vi "daqio_Write_Single.vi"(7 "daq.io Device Channel Key":string, 8 "error in (no error)":errorcluster, 9 "timestamp":timestamp, 10 "value":dbl, 11 "daq.io type in":T1={"daq.io ref"=refnum, "daq.io API Base"="http://dashboard.daq.io/api/v1", "Device Type Key"="", "Device Key"="", "Account ID"="", "online"=FALSE, "SSL"=TRUE}) -> (0 "error out":errorcluster, 3 "daq.io type out":T1={"daq.io ref"=refnum, "daq.io API Base"="http://dashboard.daq.io/api/v1", "Device Type Key"="", "Device Key"="", "Account ID"="", "online"=FALSE, "SSL"=TRUE})   [LabVIEW 2013, in "daqio minimal.lvlib"]
doc: "This VI writes a data point to a channel of a daq.io device. \n\nIf the daq.io Device Channel does not exist online, a new channel will be auto-created and data will be stored there. You have to provide a Channel Key where the value will be written to."
uses:
  daqio minimal.lvlib
  _typedefs/daqio-Type.ctl
  <vilib>/httpClient/ClientHandle.ctl
  _typedefs/daqio-TimeSeriesEntry.ctl
  _typedefs/FGV_commands.ctl
  _typedefs/daqio-Buffer-Commands.ctl
  _typedefs/connection_FGV_commands.ctl
  <vilib>/Easy HTTP Client/Easy HTTP.lvlib
  <vilib>/httpClient/LabVIEWHTTPClient.lvlib
panel:
  out "JSON string":string
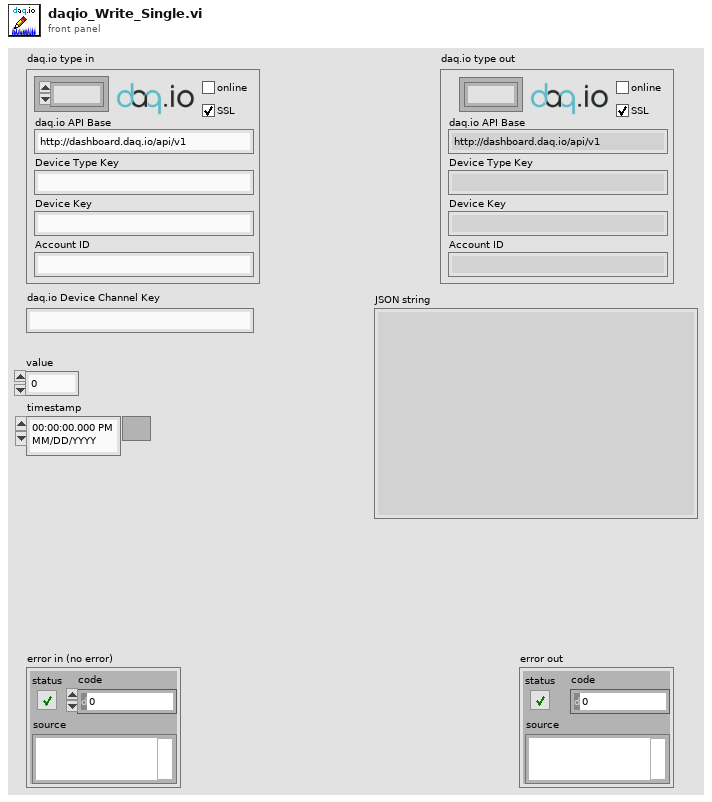
[diagram p1: front panel]
types:
  T1 = typedef "daqio minimal.lvlib/daqio-Type.ctl" = cluster{"daq.io ref":T2, "daq.io API Base":string, "Device Type Key":string, "Device Key":string, "Account ID":string, "online":bool, "SSL":bool}
  T2 = typedef "LabVIEWHTTPClient.lvlib/ClientHandle.ctl" = refnum<k1>
  T3 = typedef "daqio minimal.lvlib/FGV_commands.ctl" = enum16{"Init / Update", "Read From File", "Edit Item", "Find or Add Item", "Remove Item", "Delete All"}
  T4 = typedef "daqio minimal.lvlib/daqio-TimeSeriesEntry.ctl" = cluster{"channel_type_id":string, "device_id":string, "time":string, "value":dbl}
  T5 = typedef "daqio minimal.lvlib/daqio-Buffer-Commands.ctl" = enum16{"Add to Buffer", "Post from Buffer", "Clear Buffer", "Init"}
  T6 = typedef "daqio minimal.lvlib/connection_FGV_commands.ctl" = enum16{"Set Conn Stat", "Save Type", "Get Type from File", "Set Type", "Set Buffer", "Get"}
  T7 = typedef "daqio minimal.lvlib/daqio-Device-Type-Info-return.ctl" = cluster{"channel_types":T8[], "devices":T9[], "label":string, "event_types":T10[], "key":string, "tag_types":T11[], "id":string, "permissions":cluster{"write":string[], "read":string[]}}
  T8 = typedef "daqio minimal.lvlib/daqio-Channel-Type-POST-return.ctl" = cluster{"device_type_id":string, "id":string, "key":string, "label":string, "data_type":string, "permissions":cluster{"write":string[], "read":string[]}}
  T9 = typedef "daqio minimal.lvlib/daqio-Device.ctl" = cluster{"permissions":cluster{"write":string[], "read":string[]}, "id":string, "label":string, "key":string, "device_type_id":string, "tags":cluster{"key":string, "value":string}[], "files":string[]}
  T10 = typedef "daqio minimal.lvlib/daqio-Event-Type.ctl" = cluster{"device_type_id":string, "permissions":cluster{"read":string[], "write":string[]}, "id":string, "key":string, "label":string}
  T11 = typedef "daqio minimal.lvlib/daqio-Tag-Type-POST-return.ctl" = cluster{"label":string, "id":string, "device_type_id":string, "permissions":cluster{"write":string[], "read":string[]}, "default":string, "key":string}
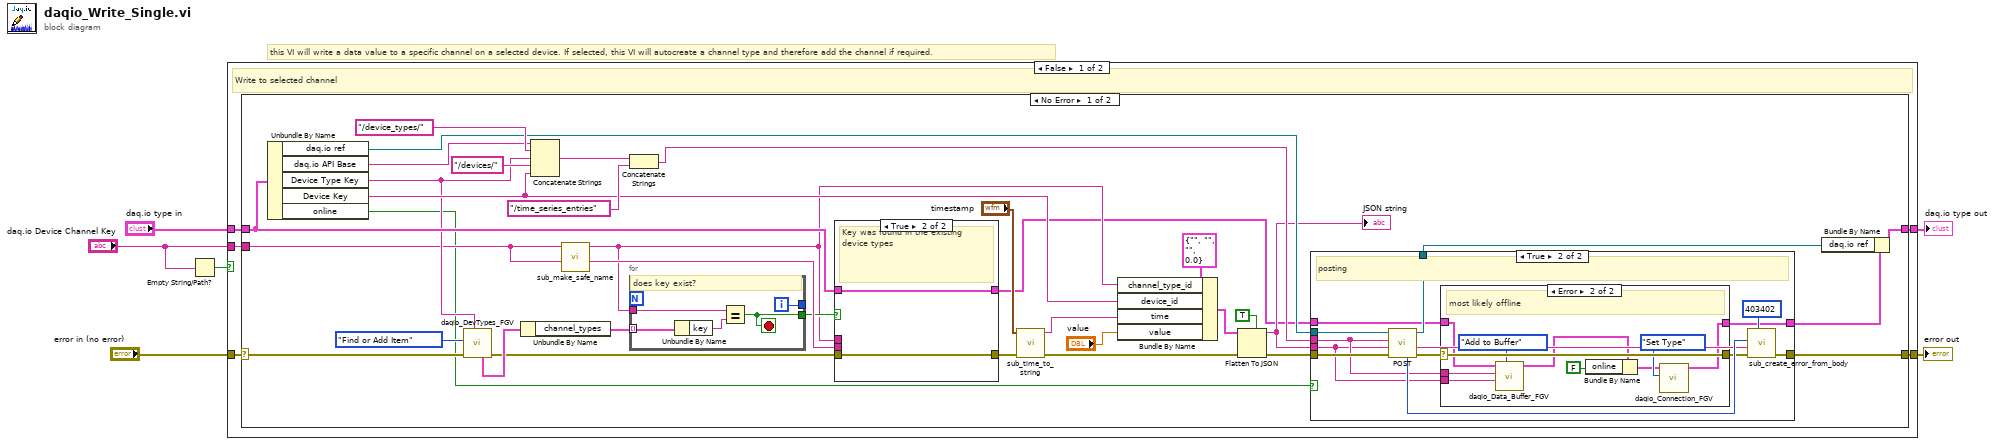
[diagram p0: block diagram]
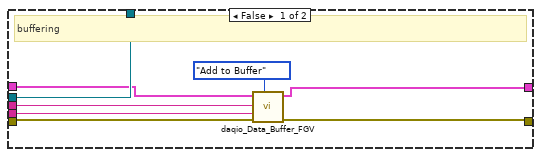
[diagram p2: hidden frame]
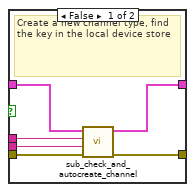
[diagram p4: hidden frame]
diagram:
  # "this VI will write a data value to a specific channel on a selected device. If selected, this VI will autocreate a channel type and therefore add the channel if required."
  n1 = Empty String/Path?(string/path="daq.io Device Channel Key") -> (empty?=w3:bool)
  n2 = case shown="False" w3 {
    tunnel: "daq.io type in" -> [w11 w95]
    tunnel: [w10 w95] -> w6
    tunnel: [w9 w94] -> w5
    tunnel: "error in (no error)" -> [w8 w94]
    tunnel: "daq.io Device Channel Key" -> [w7 _]
    frame False {
      # "Write to selected channel"
      n3 = case shown="No Error" w8 {
        selector: w8 -> [w17 w92]
        tunnel: w11 -> [w24 w93]
        tunnel: [w38 w93] -> w10
        tunnel: [w18 w92] -> w9
        tunnel: w7 -> [w22 _]
        frame No Error {
          n4 = Unbundle By Name(w24) -> ("daq.io ref"=w31:T2, "daq.io API Base"=w37:string, "Device Type Key"=w23:string, "Device Key"=w29:string, "online"=w14:bool)
          n5 = call "daqio_DevTypes_FGV.vi"("Dev Type Key"=w23, "error in (no error)"=w17, "Action"=FGV_commands."Find or Add Item") -> ("error out"=w16:errorcluster, "Dev Type out"=w26:T7)  [unwired: 4 in, 3 out]
          n6 = Unbundle By Name(w26) -> ("channel_types"=w27:T8[])
          n7 = Concatenate Strings(w37, "/device_types/", w23, "/devices/", w29) -> (w32:string)
          n8 = call "sub_make_safe_name.vi"("Input String"=w22) -> ("Safe Output String"=w15:string)  [unwired: 10 in]
          n9 = Concatenate Strings(w32, "/time_series_entries") -> (w33:string)
          n10 = for {
            tunnel: w27 -> [w91] mode=indexing
            tunnel: w15 -> [w88]
            tunnel: [w90] -> w19
            tunnel: [w89] -> _
            i -> [w89]
            stop <- w90 stop-if-true
            # "does key exist?"
            n11 = Unbundle By Name(w91) -> ("key"=w87:string)
            n12 = Equal?(x=w88, y=w87) -> (x = y?=w90:bool)
          }
          n13 = case shown="True" w19 {
            tunnel: [w84 w86] -> w13
            tunnel: [w79 w85] -> w21
            tunnel: w15 -> [w82 _]
            tunnel: w24 -> [w83 w86]
            tunnel: w22 -> [w81 _]
            tunnel: w16 -> [w80 w85]
            frame False {
              # "Create a new channel type, find the key in the local device store"
              n14 = call "sub_check_and_autocreate_channel.vi"("error in (no error)"=w80, "daq.io Device Channel Label"=w81, "daq.io Device Channel Key to write to"=w82, "daq.io type in in"=w83) -> ("error out"=w79:errorcluster, "daq.io type out"=w84:T1)  [unwired: 5 in, 1 out]
            }
            frame True {
              # "Key was found in the existing device types"
            }
          }
          n15 = call "sub_time_to_string.vi"("error in (no error)"=w21, "timestamp"="timestamp") -> ("error out"=w20:errorcluster, "time"=w41:string)  [unwired: 8 in]
          n16 = Bundle By Name(cluster=T4 {"channel_type_id"="", "device_id"="", "time"="", "value"=0.0}, "channel_type_id"=w15, "device_id"=w29, "time"=w41, "value"="value") -> (w44:T4)
          n17 = Flatten To JSON(enable LabVIEW extensions? (T)=TRUE, anything=w44, error in (no error)=w20) -> (JSON string=w30:string, 11:w45:errorcluster)
          "JSON string" <- w30
          n18 = case shown="True" w14 {
            tunnel: w45 -> [w51 w66]
            tunnel: [w53 w65] -> w35
            tunnel: w33 -> [w47 w56]
            tunnel: w31 -> [w53 w64]
            tunnel: w30 -> [w50 w55]
            tunnel: [w52 w63] -> w18
            tunnel: w13 -> [w49 w58]
            tunnel: [w48 w57] -> w12
            frame False {
              # "buffering"
              n19 = call "daqio_Data_Buffer_FGV.vi"("Buffer Command"=daqio-Buffer-Commands."Add to Buffer", "error in (no error)"=w51, "JSON Data"=w50, "API route"=w47, "daq.io type in"=w49) -> ("error out"=w52:errorcluster, "daq.io type out"=w48:T1)  [unwired: 5 in]
            }
            frame True {
              # "posting"
              n20 = call <vilib>:"POST.vi"("error in (no error)"=w66, "data"=w55, "url"=w56, "client handle"=w64) -> ("error out"=w59:errorcluster, "body"=w60:string, "client handle out"=w65:T2, "HTTP Response Code"=w62:i32)  [unwired: 3 in, 1 out]
              n21 = case shown="Error" w59 {
                selector: w59 -> [w68 w78]
                tunnel: [w68 w78] -> w54
                tunnel: [w67 w72] -> w57
                tunnel: w58 -> [w67 w71]
                tunnel: w56 -> [_ w70]
                tunnel: w55 -> [_ w69]
                frame No Error {
                }
                frame Error {
                  # "most likely offline"
                  n22 = call "daqio_Data_Buffer_FGV.vi"("Buffer Command"=daqio-Buffer-Commands."Add to Buffer", "JSON Data"=w69, "API route"=w70, "daq.io type in"=w71) -> ("daq.io type out"=w75:T1)  [unwired: 6 in, 1 out]
                  n23 = Bundle By Name(cluster=w75, "online"=FALSE) -> (w73:T1)
                  n24 = call "daqio_Connection_FGV.vi"("Enum"=connection_FGV_commands."Set Type", "daq.io type in"=w73) -> ("daq.io type out"=w72:T1)  [unwired: 6 in, 3 out]
                }
              }
              n25 = call "sub_create_error_from_body.vi"("error code"=403402, "error in (no error)"=w54, "http code"=w62, "body"=w60) -> ("error out"=w63:errorcluster)  [unwired: 7 in]
            }
          }
          n26 = Bundle By Name(cluster=w12, "daq.io ref"=w35) -> (w38:T1)
        }
        frame Error {
        }
      }
    }
    frame True {
      # "no Channel Key: nothing to do"
    }
  }
  "error out" <- w5
  "daq.io type out" <- w6
